vi "Configure Arbitrary Waveform.vi"(4 "Frequency (1000.0 Hz)":dbl, 6 "Offset (0.00 V)":dbl, 7 "Arbitrary Waveform Name (\"ARB1\")":string, 8 "error in (no error)":errorcluster, 9 "Gain (1.0 Vpp)":dbl, 10 "Channel (1: Channel1)":u16(ring) items=["Channel1", "Channel2"], 11 "VISA resource name":refnum<visa-resource-name>) -> (0 "error out":errorcluster, 3 "VISA resource name out":refnum<visa-resource-name>)   [LabVIEW 2009, in "Agilent 81150.lvlib"]
doc: "Sets the waveform parameters for an arbitrary waveform and make it the active waveform function. This VI should be called after Create Arbitrary Waveform."
uses:
  Agilent 81150.lvlib
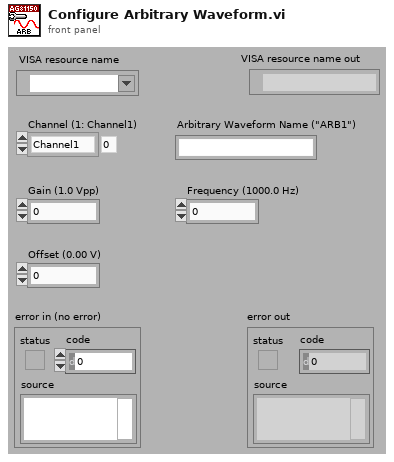
[diagram p1: front panel]
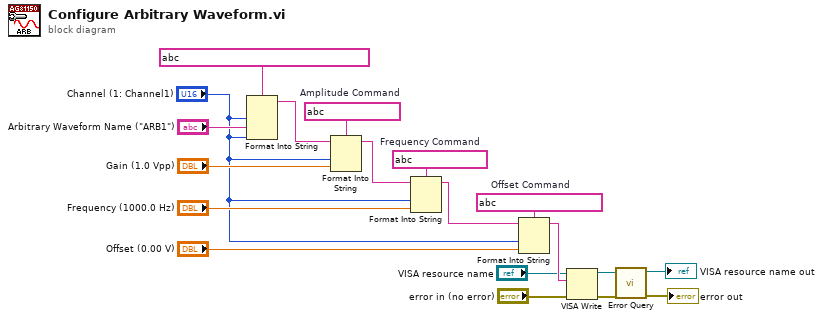
[diagram p0: block diagram]
diagram:
  w8 = string ?  # Offset Command
  w19 = string ?  # Amplitude Command
  w9 = string ?  # Frequency Command
  n1 = Format Into String(format string=string ?, "Channel (1: Channel1)", "Arbitrary Waveform Name (\"ARB1\")", "Channel (1: Channel1)") -> (resulting string=w14:string)  [unwired: 2 in, 1 out]
  n2 = Format Into String(format string=w19, initial string=w14, "Channel (1: Channel1)", "Gain (1.0 Vpp)") -> (resulting string=w18:string)  [unwired: 1 in, 1 out]
  n3 = Format Into String(format string=w9, initial string=w18, "Channel (1: Channel1)", "Frequency (1000.0 Hz)") -> (resulting string=w17:string)  [unwired: 1 in, 1 out]
  n4 = Format Into String(format string=w8, initial string=w17, "Channel (1: Channel1)", "Offset (0.00 V)") -> (resulting string=w16:string)  [unwired: 1 in, 1 out]
  n5 = VISA Write(VISA resource name="VISA resource name", write buffer=w16, error in (no error)="error in (no error)") -> (VISA resource name out=w13:refnum<visa-resource-name>, error out=w12:errorcluster)  [unwired: 1 out]
  n6 = call "Error Query.vi"("error in (no error)"=w12, "VISA resource name"=w13) -> ("error out"=→"error out":errorcluster, "VISA resource name out"=→"VISA resource name out":refnum<visa-resource-name>)  [unwired: 8 out]
